vi "Preprocessing.vi"() -> (4 "TimeStamp":dynamicdata(graph), 5 "Potência Ativa A 2":dbl[](graph), 6 "Potência Ativa A 3":dbl[](graph), 7 "Potência Ativa A":dbl[](graph))   [LabVIEW 2024]
uses:
  <vilib>/numeric/Random Number (Range) DBL.vi
panel:
  out "Potencai Ativa A 3":dbl[](array[numeric])
  out "Corrente A 3":dbl[](array[numeric])
  out "Tensão A 3":dbl[](array[numeric])
  out "Potencai Ativa A 2":dbl[](array[numeric])
  out "Corrente A 2":dbl[](array[numeric])
  out "Tensão A 2":dbl[](array[numeric])
  out "Potencai Ativa A":dbl[](array[numeric])
  out "Corrente A":dbl[](array[numeric])
  out "Tensão A":dbl[](array[numeric])
  out "Fator de potência":dbl
  in  "Limite inferior FP":dbl
  in  "Limite Superior FP":dbl=100.0
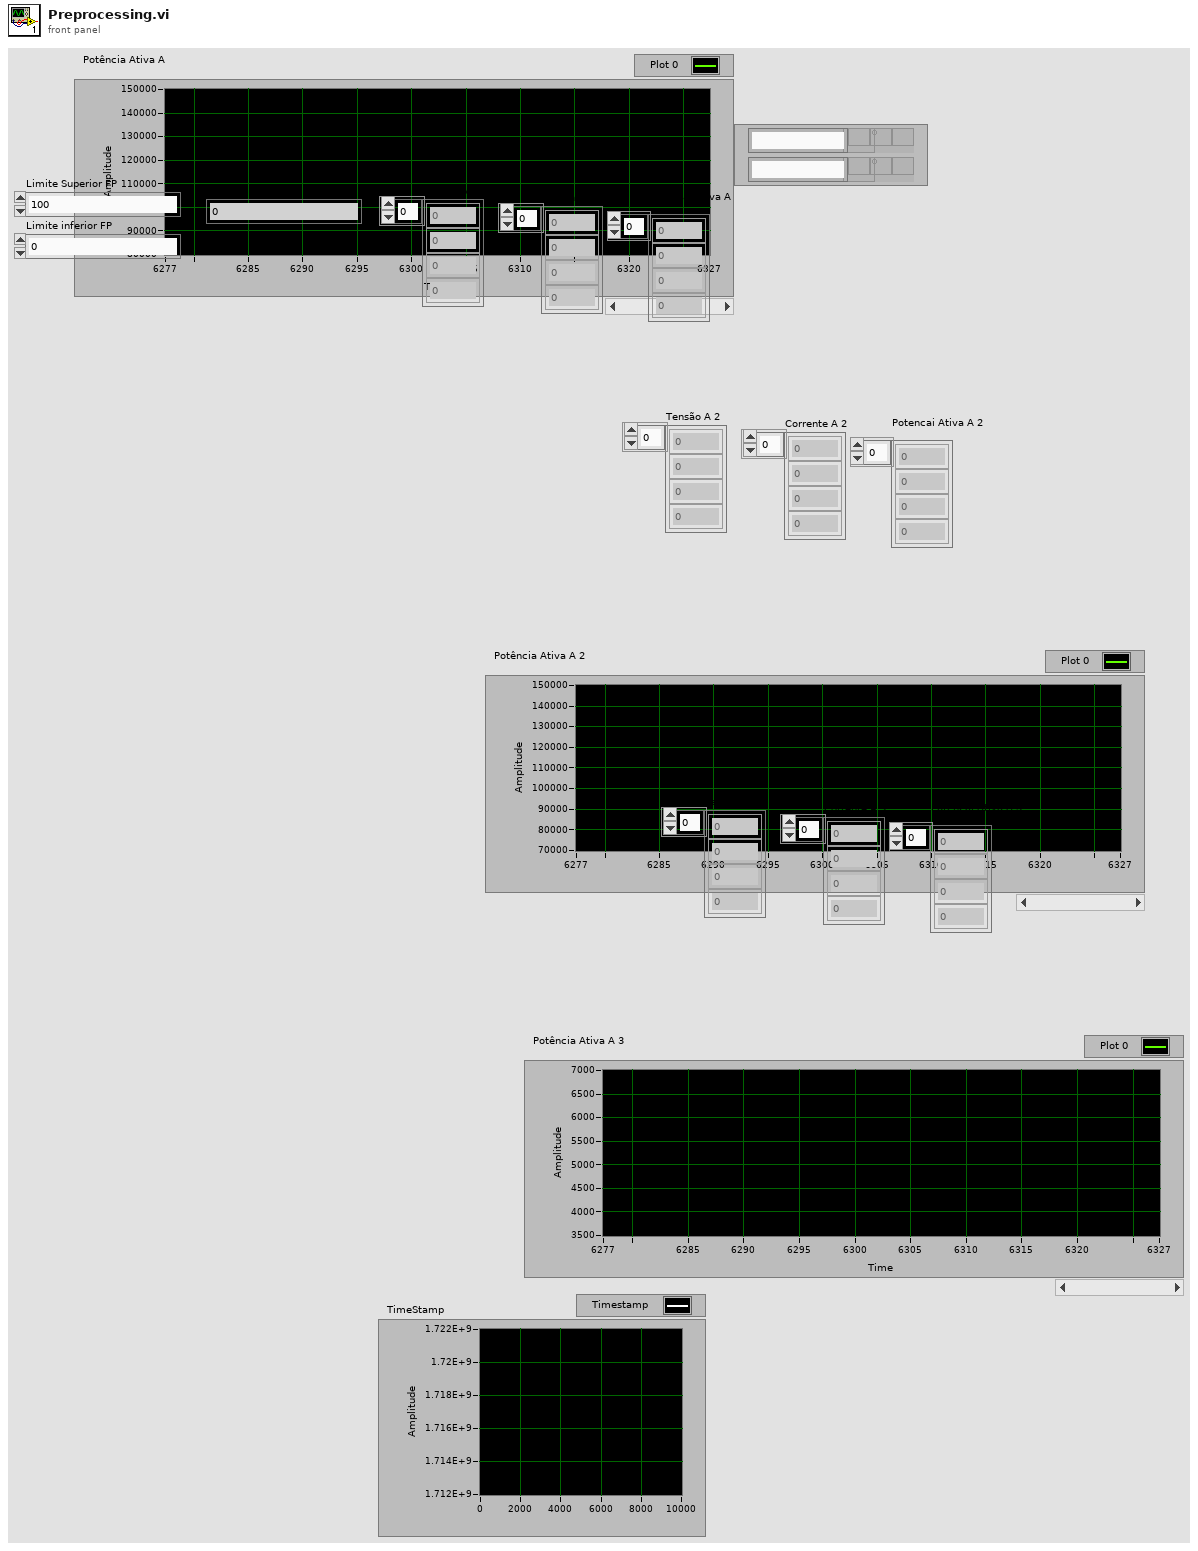
[diagram p1: front panel]
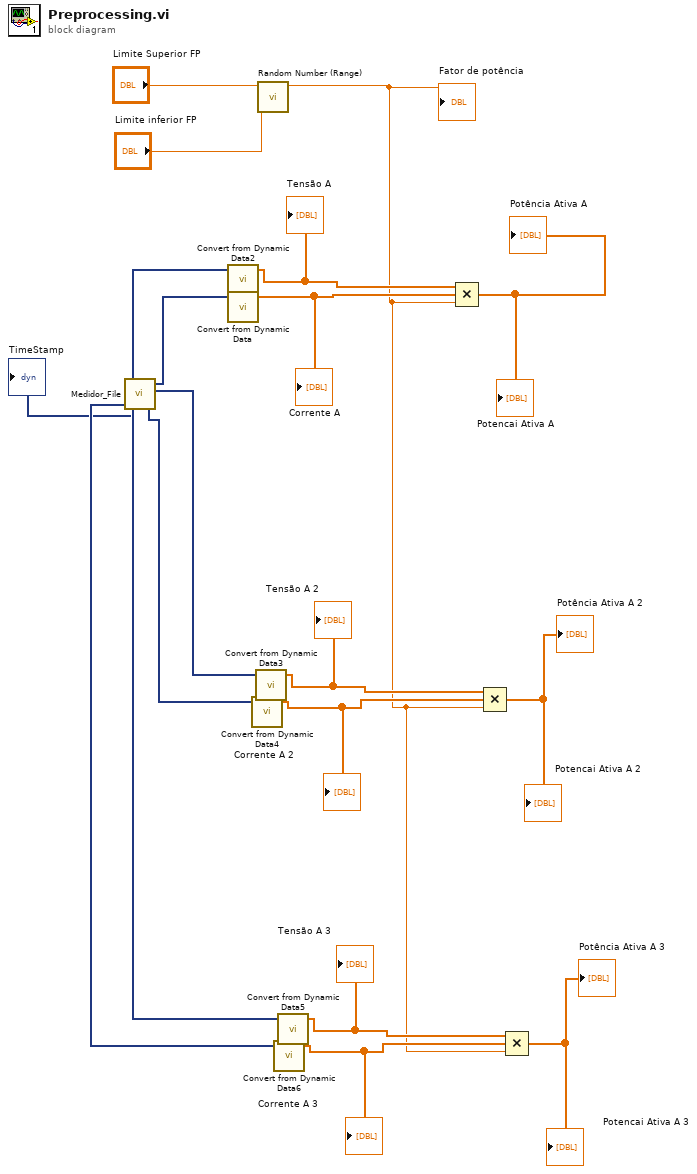
[diagram p0: block diagram]
diagram:
  n1 = call "Medidor_File.vi"() -> ("Corrente Fase C"=w3:dynamicdata, "Corrente Fase B"=w5:dynamicdata, "Corrente Fase A"=w19:dynamicdata, "TimeStamp"=→"TimeStamp":dynamicdata, "Tensão Fase C"=w2:dynamicdata, "Tensão Fase B"=w4:dynamicdata, "Tensão Fase A"=w18:dynamicdata)
  n2 = call "Convert from Dynamic Data2"("Dynamic Data Type"=w18) -> ("Array"=w17:dbl[])  [unwired: 3 in]
  "Tensão A" <- w17
  n3 = call "Convert from Dynamic Data"("Dynamic Data Type"=w19) -> ("Array"=w16:dbl[])  [unwired: 3 in]
  "Corrente A" <- w16
  n4 = call "Convert from Dynamic Data4"("Dynamic Data Type"=w5) -> ("Array"=w11:dbl[])  [unwired: 3 in]
  "Corrente A 2" <- w11
  n5 = call "Convert from Dynamic Data3"("Dynamic Data Type"=w4) -> ("Array"=w12:dbl[])  [unwired: 3 in]
  "Tensão A 2" <- w12
  n6 = call-poly <vilib>:"Random Number (Range).vi"("lower bound (0)"="Limite inferior FP", "upper bound (100)"="Limite Superior FP") -> ("number"=w6:dbl)  [unwired: 9 in]
  "Fator de potência" <- w6
  n7 = call "Convert from Dynamic Data6"("Dynamic Data Type"=w3) -> ("Array"=w8:dbl[])  [unwired: 3 in]
  "Corrente A 3" <- w8
  n8 = call "Convert from Dynamic Data5"("Dynamic Data Type"=w2) -> ("Array"=w9:dbl[])  [unwired: 3 in]
  "Tensão A 3" <- w9
  n9 = Compound Arithmetic op=MULTIPLY(w17, w16, w6) -> (→"Potência Ativa A" →"Potencai Ativa A":dbl[])
  n10 = Compound Arithmetic op=MULTIPLY(w12, w11, w6) -> (→"Potência Ativa A 2" →"Potencai Ativa A 2":dbl[])
  n11 = Compound Arithmetic op=MULTIPLY(w9, w8, w6) -> (→"Potência Ativa A 3" →"Potencai Ativa A 3":dbl[])
